vi "utility.DelayTime.vi"   [LabVIEW 2012, in "Lib_UEL.ATE.lvlib" / "Lib_App.lvlib"]
uses:
  Lib_App.lvlib
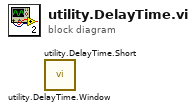
[diagram p0: block diagram]
diagram:
  n1 = call "utility.DelayTime.Window.vi"() -> ()  [unwired: 12 in]
  n2 = call "utility.DelayTime.Short.vi"() -> ()  [unwired: 12 in]
